vi "Configure Time Zone.vi"(0 "VISA resource name":refnum<visa-resource-name>, 5 "Hour (9)":i32=9 min=-13 max=13, 7 "Minute (0)":i32 min=0 max=59, 11 "error in (no error)":errorcluster) -> (4 "VISA resource name out":refnum<visa-resource-name>, 15 "error out":errorcluster)   [LabVIEW 2020, in "Yokogawa GX Series.lvlib"]
doc: "Sets the time zone.\n\nCommand: STimeZone"
uses:
  <instrlib>/Yokogawa GX Series/Yokogawa GX Series.lvlib
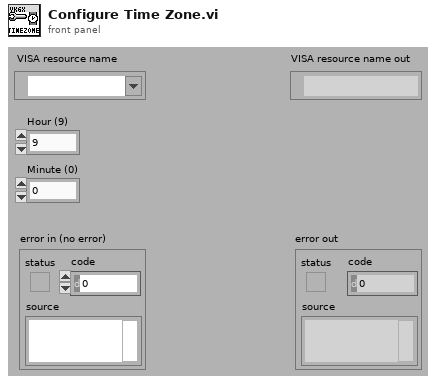
[diagram p1: front panel]
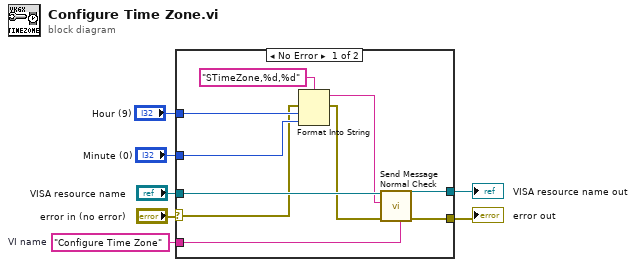
[diagram p0: block diagram]
diagram:
  w6 = "Configure Time Zone"  # VI name
  n1 = case shown="No Error" "error in (no error)" {
    selector: "error in (no error)" -> [w8 w18]
    tunnel: "VISA resource name" -> [w17 w19]
    tunnel: w6 -> [w16 _]
    tunnel: [w15 w19] -> w5
    tunnel: [w14 w18] -> w4
    tunnel: "Hour (9)" -> [w12 _]
    tunnel: "Minute (0)" -> [w11 _]
    frame No Error {
      n2 = Format Into String(format string="STimeZone,%d,%d", error in=w8, w12, w11) -> (resulting string=w9:string, error out=w10:errorcluster)  [unwired: 1 in]
      n3 = call <instrlib>:"Send Message Normal Check.vi"("Source (\"\")"=w16, "error in (no error)"=w10, "Send Message (\"\")"=w9, "VISA resource name"=w17) -> ("error out"=w14:errorcluster, "VISA resource name out"=w15:refnum<visa-resource-name>)  [unwired: 2 in, 4 out]
    }
    frame Error {
    }
  }
  "error out" <- w4
  "VISA resource name out" <- w5
